vi "Write App Configuration Path.vi"(5 "App Configuration Path":path, 9 "PythonConfiguration in":refnum<class "PythonConfiguration.lvclass">) -> (3 "PythonConfiguration out":refnum<class "PythonConfiguration.lvclass">)   [LabVIEW 2014, in "Raspberry Pi Compatible Compiler for LabVIEW.lvlib" / "PythonConfiguration.lvclass"]
uses:
  PythonConfiguration.lvclass
  PythonConfiguration.lvclass/PythonConfiguration.ctl
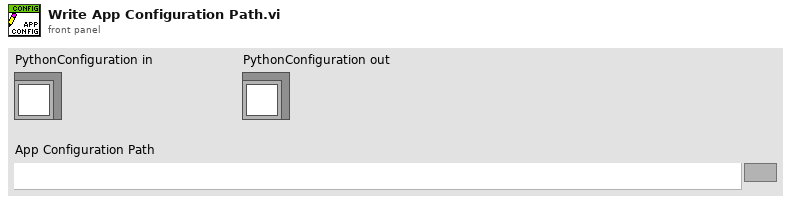
[diagram p1: front panel]
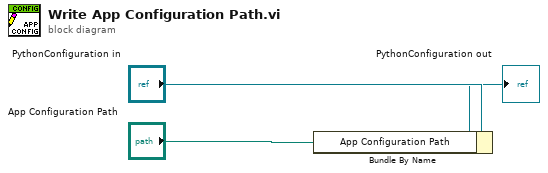
[diagram p0: block diagram]
diagram:
  n1 = Bundle By Name(cluster="PythonConfiguration in", "App Configuration Path"="App Configuration Path") -> (→"PythonConfiguration out":refnum<class "PythonConfiguration.lvclass">)
